vi "grid_adjust_z_piezo_pos.vi"(8 "Error in (no error)":errorcluster, 11 "Application ref in":refnum<vi>) -> (0 "Error out":errorcluster, 3 "Application ref out":refnum<vi>)   [LabVIEW 2014]
uses:
  <userlib>/Nanonis Prog Interface V5/Nanonis Prog Interface.lvlib
panel:
  out "Z position (m)":sgl=-1.04743926e-07 format="%#_6p"
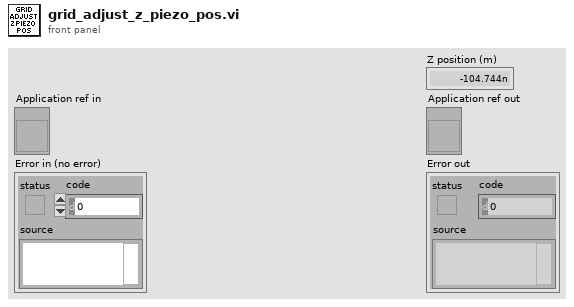
[diagram p1: front panel]
types:
  T1 = enum8{"Group 1", "Group 2", "Group 3", "Group 4", "Group 5", "Group 6"}
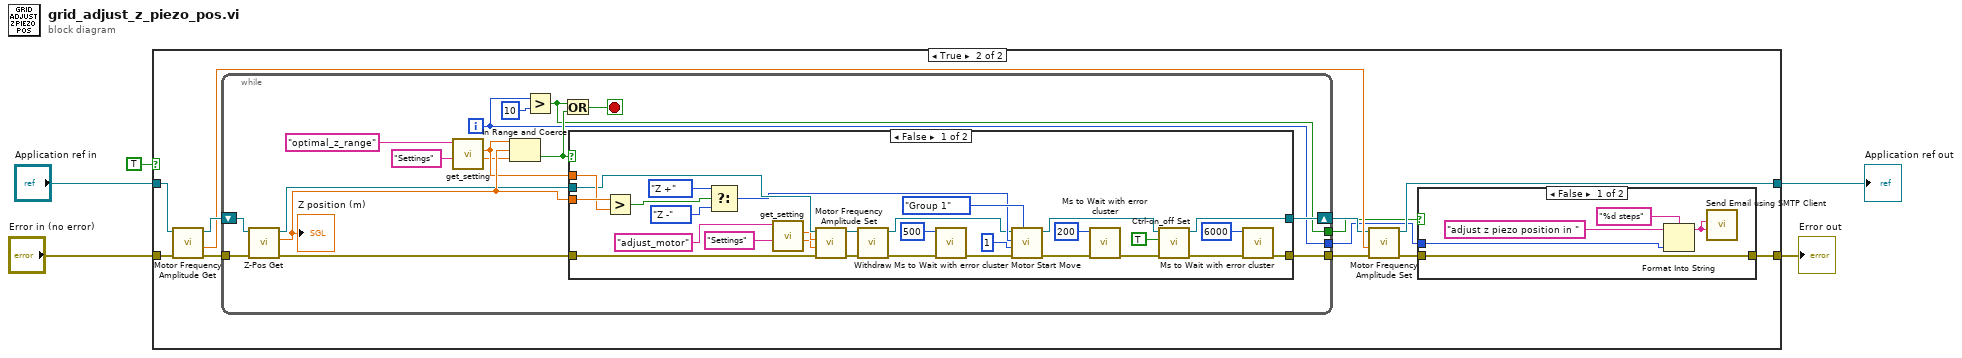
[diagram p0: block diagram]
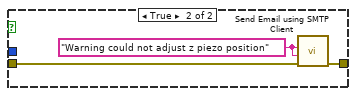
[diagram p3: hidden frame]
diagram:
  n1 = case shown="True" TRUE {
    tunnel: "Application ref in" -> [w7 w14]
    tunnel: "Error in (no error)" -> [w6 w13]
    tunnel: [w7 w12] -> w3
    tunnel: [w6 w10] -> w2
    frame False {
    }
    frame True {
      n2 = call <userlib>:"Motor Frequency Amplitude Get.vi"("Error in (no error)"=w13, "Application ref in"=w14) -> ("Error out"=w18:errorcluster, "Amplitude (V)"=w17:sgl, "Application ref out"=w19:refnum<vi>)  [unwired: 6 in, 1 out]
      n3 = while {
        tunnel: w18 -> [w40]
        shift-right: [w39] -> w16
        shift-left: w19 -> [w41]
        tunnel: [w37] -> w15
        tunnel: [w33] -> w9
        tunnel: [w28] -> w8
        i -> [w28]
        stop <- w35 stop-if-true
        n4 = call <userlib>:"Z-Pos Get.vi"("error in (no error)"=w40, "Application ref in"=w41) -> ("error out"=w36:errorcluster, "Z position (m)"=w43:sgl, "Application ref out"=w42:refnum<vi>)  [unwired: 7 in]
        "Z position (m)" <- w43
        n5 = call "get_setting.vi"("section"="Settings", "key"="optimal_z_range") -> ("output 2"=w29:dbl, "output 1"=w30:dbl)  [unwired: 5 in, 3 out]
        n6 = In Range and Coerce(upper limit=w30, x=w43, lower limit=w29) -> (In Range?=w38:bool)  [unwired: 1 out]
        n7 = Greater?(x=w28, y=10) -> (0:w33:bool)
        n8 = Or(x=w33, y=w38) -> (x .or. y?=w35:bool)
        n9 = case shown="False" w38 {
          tunnel: w43 -> [w72 _]
          tunnel: w30 -> [w71 _]
          tunnel: w42 -> [w70 w74]
          tunnel: [w54 w74] -> w39
          tunnel: [w55 w73] -> w37
          tunnel: w36 -> [w53 w73]
          frame False {
            n10 = Greater?(x=w72, y=w71) -> (0:w68:bool)
            n11 = Select(t=enum16{"X +", "X -", "Y +", "Y -", "Z +", "Z -"}."Z +" ("Direction"), s=w68, f=enum16{"X +", "X -", "Y +", "Y -", "Z +", "Z -"}."Z -" ("Direction")) -> (s? t:f=w64:enum16{"X +", "X -", "Y +", "Y -", "Z +", "Z -"})
            n12 = call "get_setting.vi"("section"="Settings", "key"="adjust_motor") -> ("output 2"=w47:dbl, "output 1"=w48:dbl)  [unwired: 5 in, 3 out]
            n13 = call <userlib>:"Motor Frequency Amplitude Set.vi"("Error in (no error)"=w53, "Amplitude (V) (NaN=no change)"=w47, "Frequency (Hz) (NaN=no change)"=w48, "Application ref in"=w70) -> ("Error out"=w52:errorcluster, "Application ref out"=w60:refnum<vi>)  [unwired: 6 in]
            n14 = call <userlib>:"Withdraw.vi"("Error in (no error)"=w52, "Application ref in"=w60) -> ("Error out"=w46:errorcluster, "Application ref out"=w63:refnum<vi>)  [unwired: 8 in]
            n15 = call <userlib>:"Ms to Wait with error cluster.vi"("error in (no error)"=w46, "milliseconds to wait"=u32 500) -> ("error out"=w45:errorcluster)  [unwired: 4 in, 1 out]
            n16 = call <userlib>:"Motor Start Move.vi"("Group"=T1."Group 1", "Error in (no error)"=w45, "Number of steps"=u16 1, "Direction"=w64, "Application ref in"=w63) -> ("Error out"=w59:errorcluster, "Application ref out"=w62:refnum<vi>)  [unwired: 4 in]
            n17 = call <userlib>:"Ms to Wait with error cluster.vi"("error in (no error)"=w59, "milliseconds to wait"=u32 200) -> ("error out"=w58:errorcluster)  [unwired: 4 in, 1 out]
            n18 = call <userlib>:"Ctrl-on_off Set.vi"("error in (no error)"=w58, "Z Controller ON/OFF"=TRUE, "Application ref in"=w62) -> ("error out"=w56:errorcluster, "Application ref out"=w54:refnum<vi>)  [unwired: 7 in]
            n19 = call <userlib>:"Ms to Wait with error cluster.vi"("error in (no error)"=w56, "milliseconds to wait"=u32 6000) -> ("error out"=w55:errorcluster)  [unwired: 4 in, 1 out]
          }
          frame True {
          }
        }
      }
      n20 = call <userlib>:"Motor Frequency Amplitude Set.vi"("Error in (no error)"=w15, "Amplitude (V) (NaN=no change)"=w17, "Application ref in"=w16) -> ("Error out"=w11:errorcluster, "Application ref out"=w12:refnum<vi>)  [unwired: 7 in]
      n21 = case shown="False" w9 {
        tunnel: w11 -> [w24 w26]
        tunnel: [w24 w25] -> w10
        tunnel: w8 -> [w21 _]
        frame False {
          n22 = Format Into String(format string="%d steps", initial string="adjust z piezo position in " ("Subject"), w21) -> (resulting string=w20:string)  [unwired: 1 in, 1 out]
          n23 = call "Send Email using SMTP Client.vi"("Message"=w20, "subject"=w20) -> ()  [unwired: 9 in, 1 out]
        }
        frame True {
          w27 = "Warning could not adjust z piezo position" ("Subject")
          n24 = call "Send Email using SMTP Client.vi"("error in (no error)"=w26, "Message"=w27, "subject"=w27) -> ("error out"=w25:errorcluster)  [unwired: 8 in]
        }
      }
    }
  }
  "Application ref out" <- w3
  "Error out" <- w2
